vi "Actor Core.vi"(8 "error in":errorcluster, 11 "HIJ Vision App IMAQdx Display In":refnum<class "HIJ Vision App IMAQdx Display.lvclass">) -> (0 "error out":errorcluster, 3 "Actor out":refnum<class "Actor.lvclass">)   [LabVIEW 2020, in "HIJ Vision App IMAQdx Display.lvlib" / "HIJ Vision App IMAQdx Display.lvclass"]
doc: "(<B>Filename</B>: Actor Framework.lvlib:Actor.lvclass:Actor Core.vi)\n\nReceives messages to the actor, reacts to them, and initiates any error handling that may shut the actor down.\n\nDescendant classes may override this VI to append parallel tasks for the actor to complete while it handles messages. Overrides use the Call Parent Method node."
uses:
  HIJ Vision App IMAQdx Display.lvclass
  HIJ Vision App IMAQdx Display.lvclass/HIJ Vision App IMAQdx Display.ctl
  <vilib>/ActorFramework/Actor/Actor.lvclass
  <vilib>/ActorFramework/Stop Msg/Stop Msg.lvclass
  Analyze/Analyze Classes/Analyze Diviation/Analyze BeamDeviation.lvclass
  Analyze/Results and Overlays/Results Beam Deviation/Analyze Results Beam Deviation.lvclass
  Analyze/Analyze Classes/Analyze Distanz/Analyze Distanz.lvclass
  Analyze/Results and Overlays/Results Distance/Analyze Results Distanz.lvclass
  Camera Actors/IMAQdx Actor/IMAQdx Actor/IMAQdx Actor.lvclass
  Application Base Actors/HIJ Vision Camera App/HIJ Vision Camera App/HIJ Vision Camera App.lvclass
  C:/POLARIS Programme/Dev LV2020/a5-beamline-cameras/Submodules/HIJ Vision/Camera Actors/Camera Actor/Camera Actor/Camera Actor.lvclass
  C:/Program Files (x86)/National Instruments/LabVIEW 2020/vi.lib/ActorFramework/Actor/Actor.lvclass
  C:/POLARIS Programme/Dev LV2020/a5-beamline-cameras/Submodules/HIJ Vision/Camera Actors/IMAQdx Actor/IMAQdx Actor/IMAQdx Actor.lvclass
  C:/POLARIS Programme/Dev LV2020/a5-beamline-cameras/Submodules/HIJ Vision/Analyze/Results and Overlays/Results Base/Analyze Results Base.lvclass
  C:/POLARIS Programme/Dev LV2020/a5-beamline-cameras/Submodules/HIJ Vision/Analyze/Results and Overlays/Results Distance/Analyze Results Distanz.lvclass
  C:/POLARIS Programme/Dev LV2020/a5-beamline-cameras/Submodules/HIJ Vision/Analyze/Results and Overlays/Results Beam Deviation/Analyze Results Beam Deviation.lvclass
  C:/POLARIS Programme/Dev LV2020/a5-beamline-cameras/Submodules/HIJ Vision/Analyze/Analyze Classes/Analyze BaseClass/Analyze BaseClass/Analyze BaseClass.lvclass
  C:/POLARIS Programme/Dev LV2020/a5-beamline-cameras/Submodules/HIJ Vision/Analyze/Analyze Classes/Analyze Diviation/Analyze BeamDeviation.lvclass
  C:/POLARIS Programme/Dev LV2020/a5-beamline-cameras/Submodules/HIJ Vision/Analyze/Analyze Classes/Analyze Distanz/Analyze Distanz.lvclass
  C:/POLARIS Programme/Dev LV2020/a5-beamline-cameras/Submodules/HIJ Vision/Application Base Actors/HIJ Vision Camera App/HIJ Vision Camera App/HIJ Vision Camera App.lvclass
  C:/POLARIS Programme/Dev LV2020/a5-beamline-cameras/Submodules/HIJ Vision/Application Base Actors/HIJ Vision Application/HIJ Vision Application/HIJ Vision Application.lvclass
  C:/POLARIS Programme/Dev LV2020/a5-beamline-cameras/Submodules/Viewable Actor/ViewableActor/ViewableActor.lvclass
  C:/POLARIS Programme/Dev LV2020/a5-beamline-cameras/Submodules/HIJ Vision/Analyze/Analyze Actor/IAnalysis/IAnalysis.lvclass
  C:/POLARIS Programme/Dev LV2020/a5-beamline-cameras/Submodules/HIJ Vision/Camera Actors/Camera Actor/ICamera/ICamera.lvclass
  C:/POLARIS Programme/Dev LV2020/a5-beamline-cameras/Submodules/HIJ Vision/User Applications/HIJ Vision App IMAQdx Display/HIJ Vision App IMAQdx Display/HIJ Vision App IMAQdx Display.lvclass
  Viewable Actor/ViewableActor Messages/Proceed Menu Selection Msg/Proceed Menu Selection Msg.lvclass
panel:
  in  "Stop Button":bool
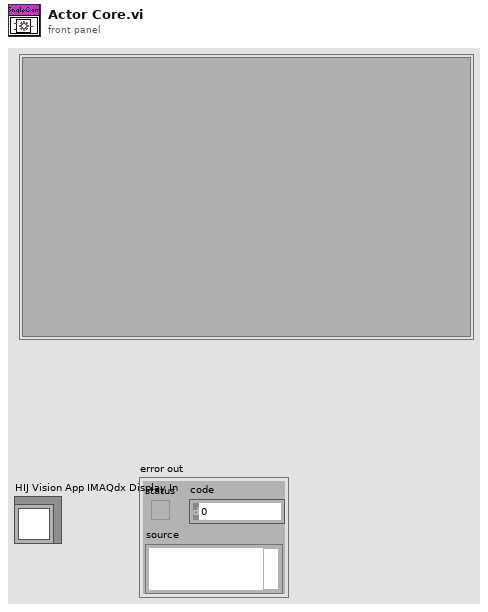
[diagram p1: front panel]
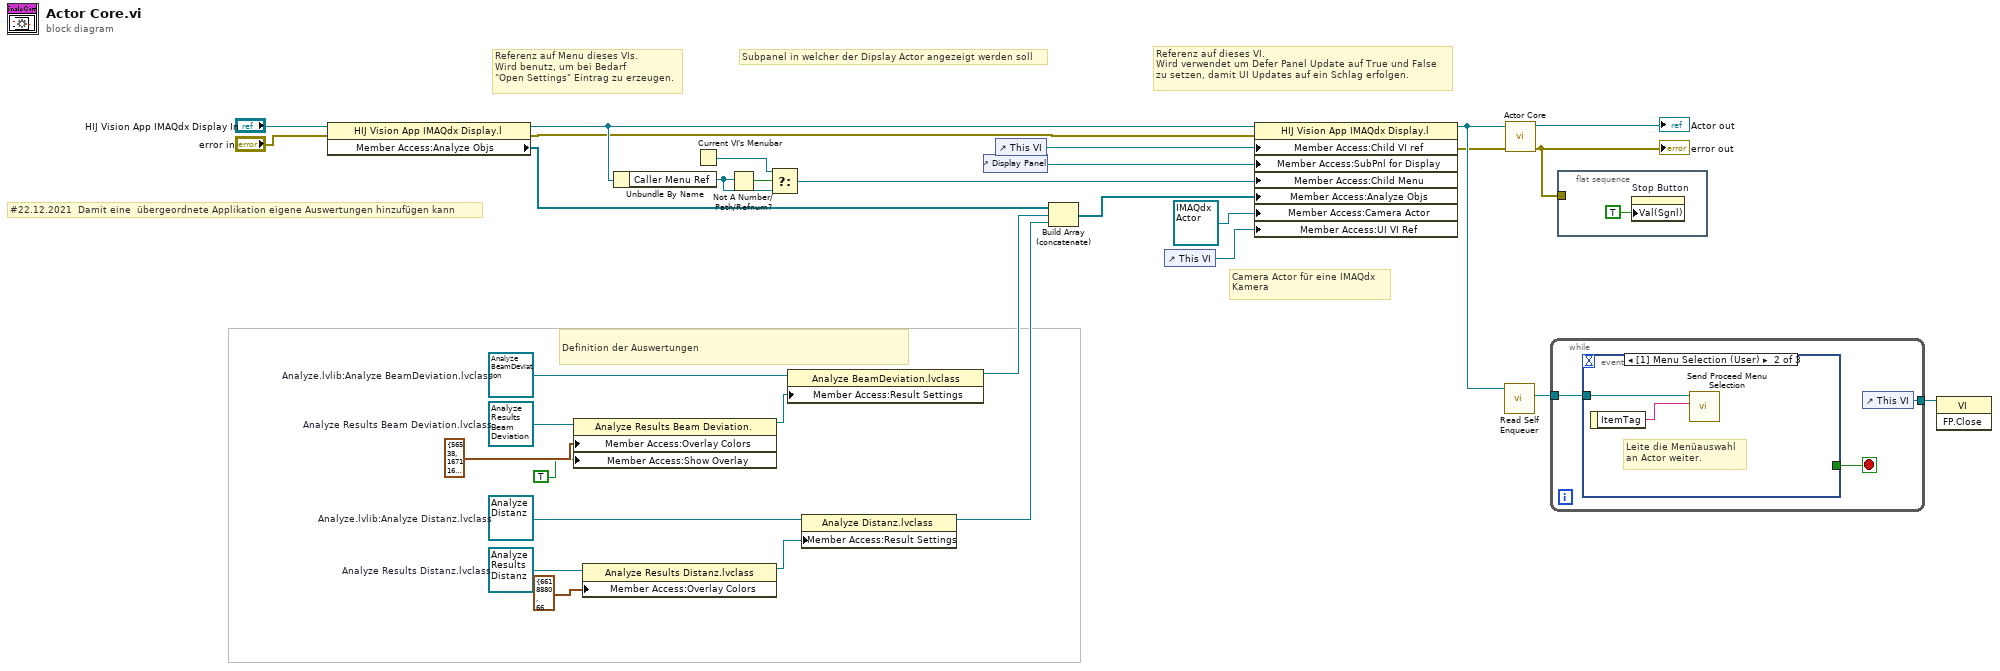
[diagram p0: block diagram]
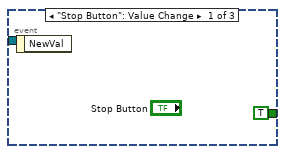
[diagram p2: hidden frame]
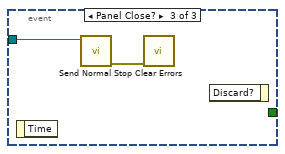
[diagram p3: hidden frame]
diagram:
  w24 = refnum<class "Analyze Results Distanz.lvclass"> refnum  # Analyze Results Distanz.lvclass
  w25 = refnum<class "Analyze Distanz.lvclass"> refnum  # Analyze.lvlib:Analyze Distanz.lvclass
  w27 = refnum<class "Analyze Results Beam Deviation.lvclass"> refnum  # Analyze Results Beam Deviation.lvclass
  w28 = refnum<class "Analyze BeamDeviation.lvclass"> refnum  # Analyze.lvlib:Analyze BeamDeviation.lvclass
  # "#22.12.2021  Damit eine  übergeordnete Applikation eigene Auswertungen hinzufügen kann"
  # "Camera Actor für eine IMAQdx\nKamera"
  # "Referenz auf Menu dieses VIs.\nWird benutz, um bei Bedarf \n\"Open Settings\" Eintrag zu erzeugen."
  # "Referenz auf dieses VI.\nWird verwendet um Defer Panel Update auf True und False\nzu setzen, damit UI Updates auf ein Schlag erfolgen."
  # "Definition der Auswertungen"
  # "Subpanel in welcher der Dipslay Actor angezeigt werden soll"
  n1 = property class="HIJ Vision App IMAQdx Display.l"(reference="HIJ Vision App IMAQdx Display In", error in="error in") -> (reference out=w4:refnum<class "HIJ Vision App IMAQdx Display.lvclass">, error out=w2:errorcluster, "Member Access:Analyze Objs"=w1:refnum<class "Analyze BaseClass.lvclass">[])
  n2 = property class="Analyze Results Beam Deviation."(reference=w27, "Member Access:Overlay Colors"=cluster{"Border":u32, "Text":u32} {"Border"=56538, "Text"=16711680} ("Colors"), "Member Access:Show Overlay"=TRUE ("Show Overlay")) -> (reference out=w15:refnum<class "Analyze Results Beam Deviation.lvclass">)  [unwired: 1 in, 1 out]
  n3 = property class="Analyze Results Distanz.lvclass"(reference=w24, "Member Access:Overlay Colors"=cluster{"Border":u32, "Text":u32} {"Border"=6618880, "Text"=6618880} ("Colors")) -> (reference out=w14:refnum<class "Analyze Results Distanz.lvclass">)  [unwired: 1 in, 1 out]
  n4 = Unbundle By Name(w4) -> ("Caller Menu Ref"=w8:refnum<k9>)
  n5 = Current VI's Menubar() -> (w9:refnum<k9>)
  n6 = Not A Number/Path/Refnum?(number/path/refnum=w8) -> (NaN/Path/Refnum?=w11:bool)
  n7 = Select(t=w9, s=w11, f=w8) -> (s? t:f=w10:refnum<k9>)
  n8 = property class="Analyze BeamDeviation.lvclass"(reference=w28, "Member Access:Result Settings"=w15) -> (reference out=w16:refnum<class "Analyze BeamDeviation.lvclass">)  [unwired: 1 in, 1 out]
  n9 = property class="Analyze Distanz.lvclass"(reference=w25, "Member Access:Result Settings"=w14) -> (reference out=w13:refnum<class "Analyze Distanz.lvclass">)  [unwired: 1 in, 1 out]
  n10 = control-ref of="Display Panel"() -> (w18:refnum<vi>)
  n11 = control-ref of="This VI"() -> (w21:refnum<vi>)
  n12 = Build Array (concatenate)(w1, w16, w13) -> (w19:refnum<class "Analyze BaseClass.lvclass">[])
  n13 = control-ref of="This VI"() -> (w12:refnum<vi>)
  n14 = property class="HIJ Vision App IMAQdx Display.l"(reference=w4, error in=w2, "Member Access:Child VI ref"=w21, "Member Access:SubPnl for Display"=w18, "Member Access:Child Menu"=w10, "Member Access:Analyze Objs"=w19, "Member Access:Camera Actor"=refnum<class "IMAQdx Actor.lvclass"> refnum ("IMAQdx Actor.lvlib:IMAQdx Actor.lvclass"), "Member Access:UI VI Ref"=w12) -> (reference out=w22:refnum<class "HIJ Vision App IMAQdx Display.lvclass">, error out=w20:errorcluster)
  n15 = call <vilib>:"Read Self Enqueuer.vi"("Actor"=w22) -> ("Self Enqueuer"=w29:refnum<class "Message Enqueuer.lvclass">)  [unwired: 10 in]
  n16 = call-parent "Actor Core.vi"("error in"=w20, "HIJ Vision Camera App In"=w22) -> ("error out"=w30:errorcluster, "Actor out"=→"Actor out":refnum<class "Actor.lvclass">)  [unwired: 8 in]
  "error out" <- w30
  n17 = while {
    tunnel: w29 -> [w33]
    tunnel: [w32] -> w6
    stop <- w34 stop-if-true
    n18 = event shown="[1] Menu Selection (User)" {
      selector: _ -> [_ _ _]
      dyn-events: _ -> [_ _ _]
      timeout: _ -> [_ _ _]
      tunnel: [TRUE _ _] -> w34
      tunnel: w33 -> [_ w36 w39]
      event "Stop Button": Value Change {
        n19 = event-data() -> ()  [unwired: 1 in, 1 out]
      }
      event Menu Selection (User) {
        # "Leite die Menüauswahl \nan Actor weiter."
        n20 = event-data() -> ("ItemTag"=w37:string)  [unwired: 1 in]
        n21 = call "Send Proceed Menu Selection.vi"("Menu Tag"=w37, "Message Enqueuer"=w36) -> ()  [unwired: 8 in, 2 out]
      }
      event Panel Close? {
        n22 = event-data() -> ()  [unwired: 1 in, 1 out]
        n23 = call <vilib>:"Send Normal Stop.vi"("Message Enqueuer"=w39) -> ("error out"=w38:errorcluster)  [unwired: 10 in]
        n24 = call <vilib>:"Clear Errors.vi"("error in (no error)"=w38) -> ()  [unwired: 5 in, 2 out]
        n25 = event-data() -> ()  [unwired: 2 in, 1 out]
      }
    }
    n26 = control-ref of="This VI"() -> (w32:refnum<vi>)
  }
  n27 = flat-sequence {
    tunnel: w30 -> [_]
    frame #0 {
      n28 = property on="Stop Button" class="Bool (strict)"("Val(Sgnl)"=TRUE) -> ()  [unwired: 2 in, 2 out]
    }
  }
  n29 = invoke class="VI" method="FP.Close"(reference=w6) -> ()  [unwired: 2 in, 3 out]
